vi "AODInterfaceQueue.vi"() -> ()   [LabVIEW 2015, in "AODControl.lvlib"]
uses:
  MessageQueue/QueueOperations/All Message Queues.ctl
  MessageQueue/QueueOperations/Message Cluster.ctl
  AODControl.lvlib
  MessageQueue/MessageQueue.lvlib
panel:
  out "AOD Interface Queue":T1
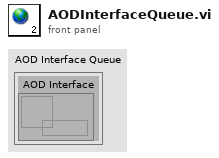
[diagram p1: front panel]
types:
  T1 = typedef "AODControl.lvlib/MessageQueue.lvlib/All Message Queues.ctl" = cluster{" AOD Interface":refnum<queue>}
diagram:
